vi "Append to log (SubVI).vi"(1 "log length":i32=10000, 2 "to append":string, 3 "log in":string) -> (0 "log out":string)   [LabVIEW 2016]
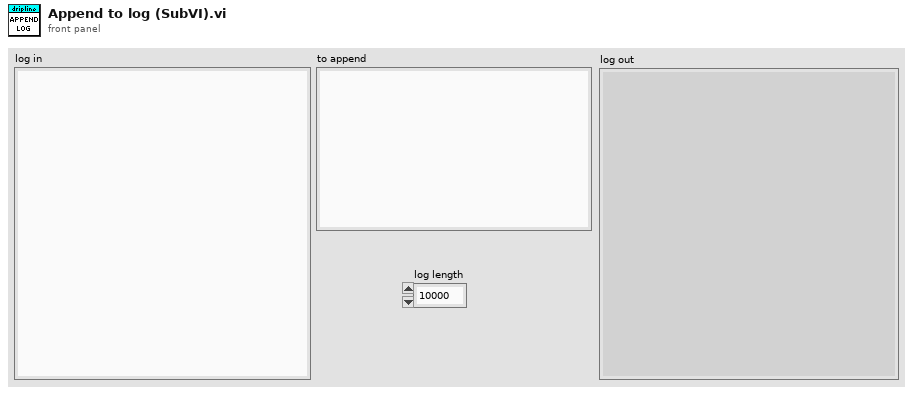
[diagram p1: front panel]
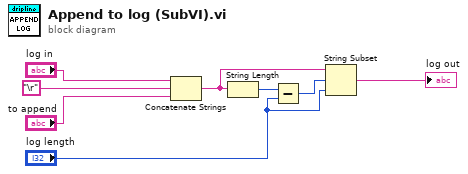
[diagram p0: block diagram]
diagram:
  n1 = Concatenate Strings("log in", "\r", "to append") -> (w5:string)
  n2 = String Length(string=w5) -> (length=w6:i32)
  n3 = Subtract(x=w6, y="log length") -> (x-y=w7:i32)
  n4 = String Subset(string=w5, offset (0)=w7, length (rest)="log length") -> (substring=→"log out":string)
